vi "post_processing.vi"(4 "wl end":dbl, 6 "wl start":dbl, 7 "Phase warning":dbl, 8 "Wavelengths":dbl[](array[numeric]), 9 "Phase in (r=wl, c=v)":dbl[][](array[numeric]), 10 "Zeroes (idx)":cluster{"Splice indices":i32[]}[](array[cluster]), 11 "Extrapolate":bool) -> (0 "Phase out (r=wl, c=v)":dbl[][](array[numeric]), 3 "Errors":T1)   [LabVIEW 2019]
uses:
  <vilib>/gmath/NI_Gmath.lvlib
panel:
  out "max 2nd deriv":dbl
  out "d2/dV2 Phase":dbl[](array[numeric])
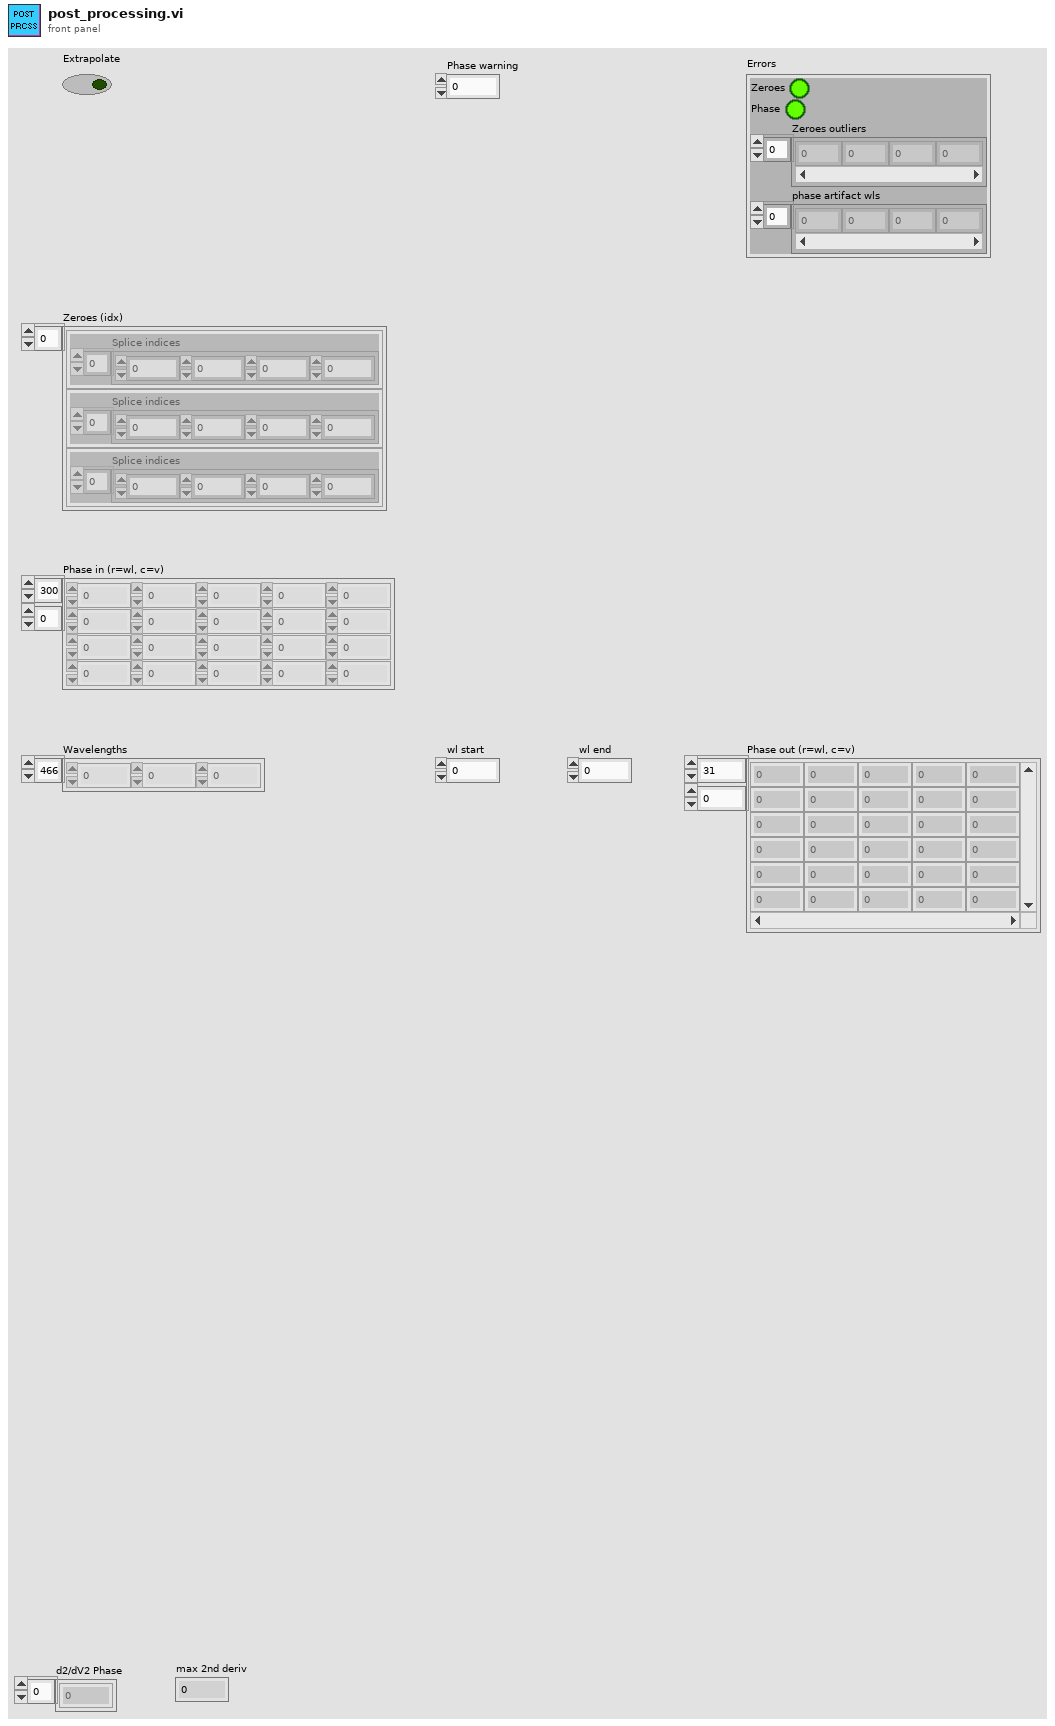
[diagram p1: front panel]
types:
  T1 = cluster{"Zeroes":bool, "Phase":bool, "Zeroes outliers":dbl[], "phase artifact wls":dbl[]}
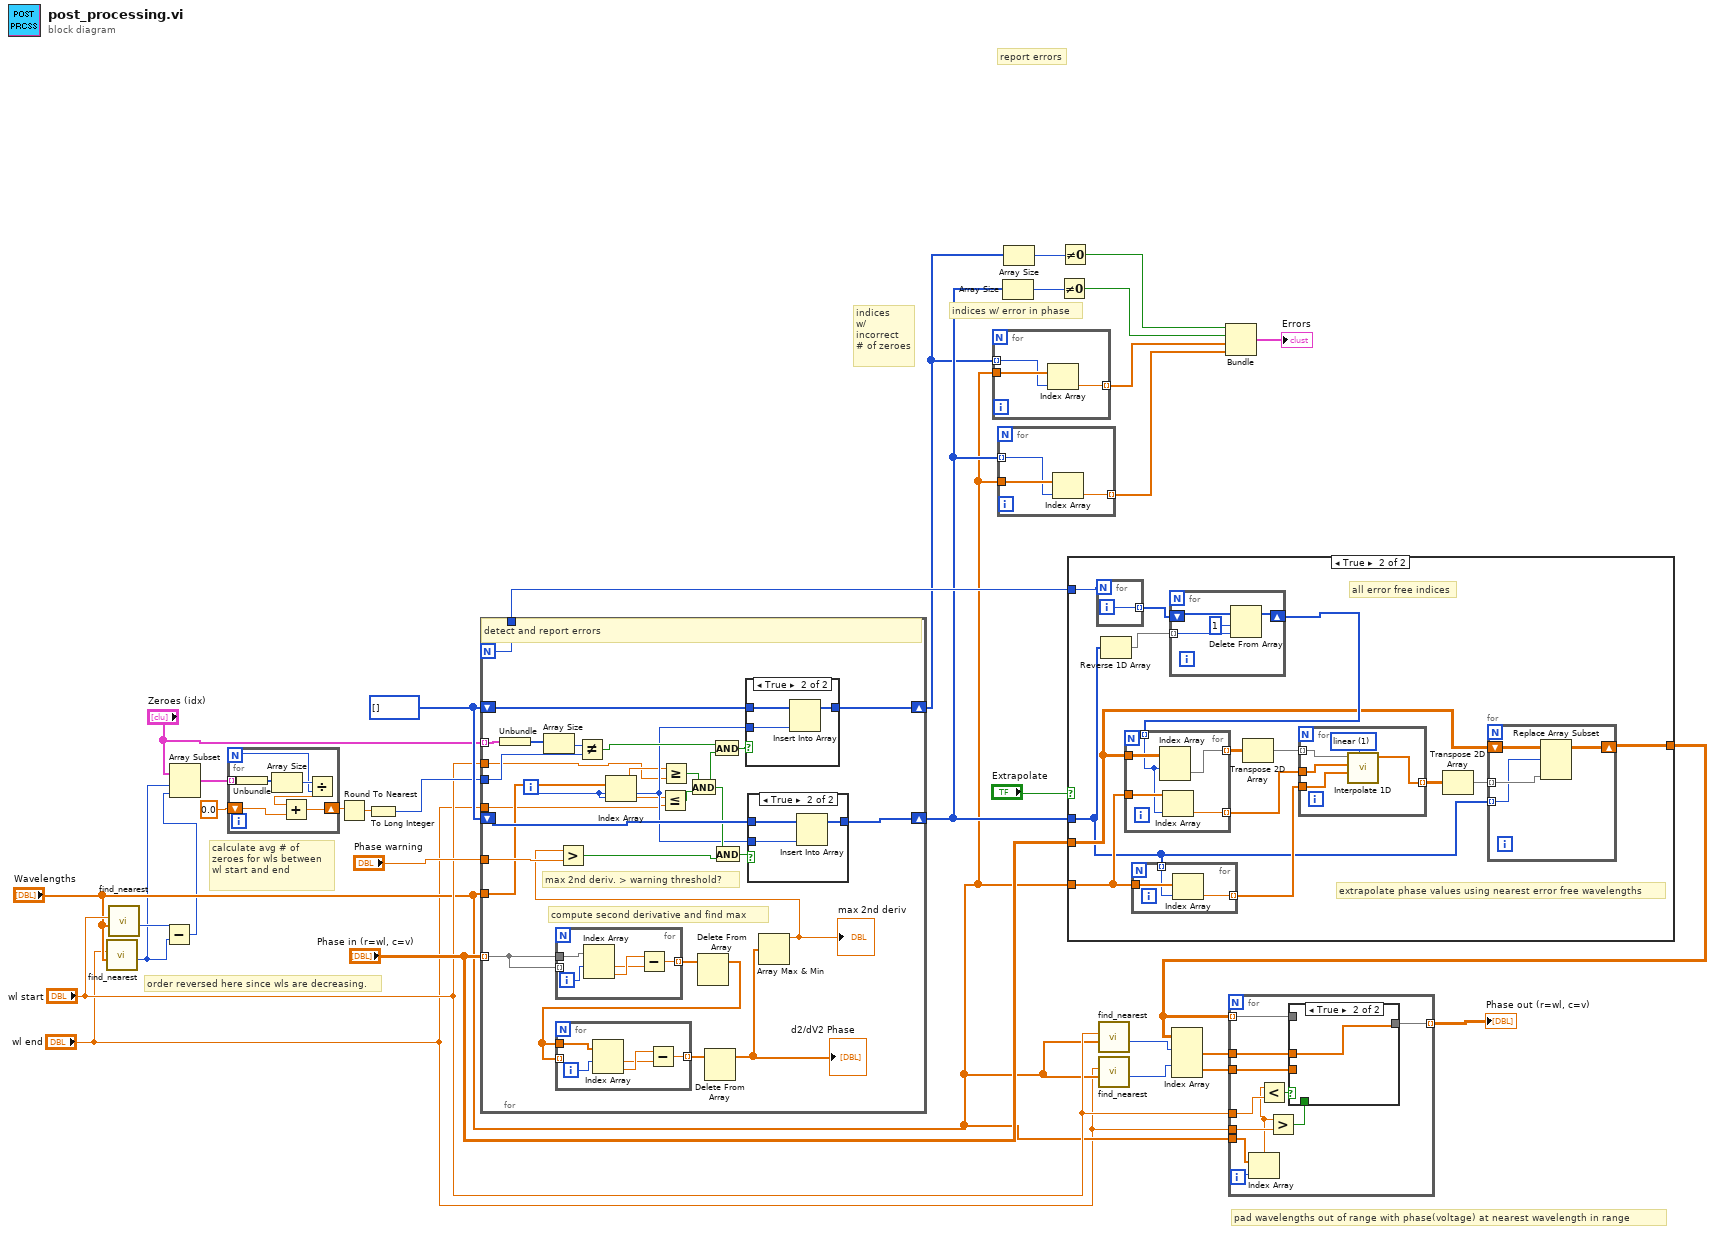
[diagram p0: block diagram]
diagram:
  w32 = i32[] []
  # "calculate avg # of zeroes for wls between wl start and end"
  # "order reversed here since wls are decreasing."
  # "indices w/ error in phase"
  # "indices\nw/\nincorrect\n# of zeroes"
  # "report errors"
  # "pad wavelengths out of range with phase(voltage) at nearest wavelength in range"
  n1 = call "find_nearest.vi"("Sorted Array (<)"="Wavelengths", "Key"="wl end") -> ("Nearest index"=w2:i32)  [unwired: 6 in, 3 out]
  n2 = call "find_nearest.vi"("Sorted Array (<)"="Wavelengths", "Key"="wl start") -> ("Nearest index"=w3:i32)  [unwired: 6 in, 3 out]
  n3 = Subtract(x=w3, y=w2) -> (x-y=w1:i32)
  n4 = Array Subset(array="Zeroes (idx)", index=w2, length=w1) -> (w5:cluster{"Splice indices":i32[]}[])
  n5 = for {
    N -> [w36]
    tunnel: w5 -> [w38] mode=indexing
    shift-right: [w33] -> w11
    shift-left: 0.0 -> [w35]
    n6 = Unbundle(w38) -> ("Splice indices"=w39:i32[])
    n7 = Array Size(array=w39) -> (size(s)=w37:i32)
    n8 = Divide(x=w37, y=w36) -> (x/y=w34:dbl)
    n9 = Add(x=w34, y=w35) -> (x+y=w33:dbl)
  }
  n10 = Round To Nearest(number=w11) -> (nearest integer value=w10:dbl)
  n11 = To Long Integer(number=w10) -> (32bit integer=w9:i32)
  n12 = for {
    N -> [w54]
    shift-right: [w66] -> w22
    shift-left: w32 -> [w67]
    shift-right: [w63] -> w21
    shift-left: w32 -> [w64]
    tunnel: w9 -> [w62]
    tunnel: "Phase warning" -> [w61]
    tunnel: "Zeroes (idx)" -> [w43] mode=indexing
    tunnel: "Phase in (r=wl, c=v)" -> [w57] mode=indexing
    tunnel: [w54] -> w29
    tunnel: "Wavelengths" -> [w45]
    tunnel: "wl start" -> [w41]
    tunnel: "wl end" -> [w40]
    i -> [w46]
    # "max 2nd deriv. > warning threshold?"
    # "compute second derivative and find max"
    # "detect and report errors"
    n13 = Unbundle(w43) -> ("Splice indices"=w42:i32[])
    n14 = Array Size(array=w42) -> (size(s)=w65:i32)
    n15 = for {
      tunnel: w57 -> [w75]
      tunnel: [w73] -> w58 mode=indexing
      tunnel: w57 -> [_] mode=indexing
      i -> [w77]
      n16 = Index Array(array=w75, index #1=w77) -> (element #1=w74:dbl, element #2=w76:dbl)  [unwired: 1 in]
      n17 = Subtract(x=w76, y=w74) -> (x-y=w73:dbl)
    }
    n18 = Not Equal?(x=w65, y=w62) -> (x != y?=w51:bool)
    n19 = Index Array(array=w45, index=w46) -> (element=w44:dbl)
    n20 = Less Or Equal?(x=w44, y=w40) -> (x <= y?=w53:bool)
    n21 = Greater Or Equal?(x=w44, y=w41) -> (x >= y?=w52:bool)
    n22 = And(x=w52, y=w53) -> (x .and. y?=w47:bool)
    n23 = Delete From Array(array=w58) -> (array with subset deleted=w56:dbl[])  [unwired: 2 in, 1 out]
    n24 = for {
      tunnel: w56 -> [w70]
      tunnel: [w68] -> w59 mode=indexing
      tunnel: w56 -> [_] mode=indexing
      i -> [w72]
      n25 = Index Array(array=w70, index #1=w72) -> (element #1=w69:dbl, element #2=w71:dbl)  [unwired: 1 in]
      n26 = Subtract(x=w71, y=w69) -> (x-y=w68:dbl)
    }
    n27 = Delete From Array(array=w59) -> (array with subset deleted=w60:dbl[])  [unwired: 2 in, 1 out]
    "d2/dV2 Phase" <- w60
    n28 = And(x=w51, y=w47) -> (x .and. y?=w50:bool)
    n29 = case shown="True" w50 {
      tunnel: w46 -> [_ w80]
      tunnel: w64 -> [w78 w81]
      tunnel: [w78 w79] -> w63
      frame False {
      }
      frame True {
        n30 = Insert Into Array(array=w81, new element=w80) -> (w79:i32[])  [unwired: 1 in]
      }
    }
    n31 = Array Max & Min(array=w60) -> (max value=w55:dbl)  [unwired: 3 out]
    "max 2nd deriv" <- w55
    n32 = Greater?(x=w55, y=w61) -> (0:w49:bool)
    n33 = And(x=w47, y=w49) -> (x .and. y?=w48:bool)
    n34 = case shown="True" w48 {
      tunnel: w46 -> [_ w84]
      tunnel: w67 -> [w82 w85]
      tunnel: [w82 w83] -> w66
      frame False {
      }
      frame True {
        n35 = Insert Into Array(array=w85, new element=w84) -> (w83:i32[])  [unwired: 1 in]
      }
    }
  }
  n36 = for {
    tunnel: w21 -> [w87] mode=indexing
    tunnel: "Wavelengths" -> [w88]
    tunnel: [w86] -> w18 mode=indexing
    n37 = Index Array(array=w88, index=w87) -> (element=w86:dbl)
  }
  n38 = for {
    tunnel: w22 -> [w90] mode=indexing
    tunnel: "Wavelengths" -> [w91]
    tunnel: [w89] -> w17 mode=indexing
    n39 = Index Array(array=w91, index=w90) -> (element=w89:dbl)
  }
  n40 = Array Size(array=w22) -> (size(s)=w24:i32)
  n41 = Array Size(array=w21) -> (size(s)=w23:i32)
  n42 = Not Equal To 0?(x=w24) -> (x != 0?=w19:bool)
  n43 = Not Equal To 0?(x=w23) -> (x != 0?=w20:bool)
  n44 = case shown="True" "Extrapolate" {
    tunnel: "Phase in (r=wl, c=v)" -> [w92 w98]
    tunnel: [w92 w95] -> w15
    tunnel: w29 -> [_ w106]
    tunnel: w22 -> [_ w96]
    tunnel: "Wavelengths" -> [_ w103]
    frame False {
    }
    frame True {
      # "extrapolate phase values using nearest error free wavelengths"
      # "all error free indices"
      n45 = for {
        N: w106 -> [_]
        tunnel: [w111] -> w94 mode=indexing
        i -> [w111]
      }
      n46 = Reverse 1D Array(array=w96) -> (reversed array=w93:i32[])
      n47 = for {
        tunnel: w103 -> [w123]
        tunnel: [w122] -> w100 mode=indexing
        tunnel: w96 -> [w121] mode=indexing
        n48 = Index Array(array=w123, index=w121) -> (element=w122:dbl)
      }
      n49 = for {
        shift-right: [w109] -> w105
        shift-left: w94 -> [w110]
        tunnel: w93 -> [w108] mode=indexing
        n50 = Delete From Array(array=w110, length=1, index=w108) -> (array with subset deleted=w109:i32[])  [unwired: 1 out]
      }
      n51 = for {
        tunnel: w98 -> [w128]
        tunnel: w105 -> [w125] mode=indexing
        tunnel: [w127] -> w104 mode=indexing
        tunnel: w103 -> [w126]
        tunnel: [w124] -> w101 mode=indexing
        n52 = Index Array(array=w128, index (row)=w125) -> (element=w127:dbl[])  [unwired: 1 in]
        n53 = Index Array(array=w126, index=w125) -> (element=w124:dbl)
      }
      n54 = Transpose 2D Array(2D array=w104) -> (transposed array=w102:dbl[][])
      n55 = for {
        tunnel: w102 -> [w120] mode=indexing
        tunnel: w101 -> [w119]
        tunnel: w100 -> [w118]
        tunnel: [w116] -> w99 mode=indexing
        w117 = 1 items=["nearest", "linear", "spline", "cubic Hermite", "Lagrange"] ("method")
        n56 = call <vilib>:"Interpolate 1D.vi"("method"=w117, "xi"=w118, "X"=w119, "Y"=w120) -> ("yi"=w116:dbl[])  [unwired: 5 in, 2 out]
      }
      n57 = Transpose 2D Array(2D array=w99) -> (transposed array=w97:dbl[][])
      n58 = for {
        tunnel: w97 -> [w114] mode=indexing
        tunnel: w96 -> [w113] mode=indexing
        shift-right: [w112] -> w95
        shift-left: w98 -> [w115]
        n59 = Replace Array Subset(array=w115, new element=w114, index (row)=w113) -> (w112:dbl[][])  [unwired: 1 in]
      }
    }
  }
  n60 = call "find_nearest.vi"("Sorted Array (<)"="Wavelengths", "Key"="wl start") -> ("Nearest index"=w13:i32)  [unwired: 6 in, 3 out]
  n61 = call "find_nearest.vi"("Sorted Array (<)"="Wavelengths", "Key"="wl end") -> ("Nearest index"=w14:i32)  [unwired: 6 in, 3 out]
  n62 = Index Array(array=w15, index (row) #1=w13, index (row) #2=w14) -> (element #1=w27:dbl[], element #2=w26:dbl[])  [unwired: 2 in]
  n63 = Bundle(w20, w19, w18, w17) -> (→"Errors":cluster{bool, bool, dbl[], dbl[]})  [unwired: 1 in]
  n64 = for {
    tunnel: w15 -> [w133] mode=indexing
    tunnel: "wl start" -> [w139]
    tunnel: "wl end" -> [w137]
    tunnel: w27 -> [w135]
    tunnel: w26 -> [w134]
    tunnel: [w132] -> w25 mode=indexing
    tunnel: "Wavelengths" -> [w131]
    i -> [w130]
    n65 = Index Array(array=w131, index=w130) -> (element=w129:dbl)
    n66 = Less?(x=w129, y=w139) -> (x < y?=w138:bool)
    n67 = Greater?(x=w129, y=w137) -> (0:w136:bool)
    n68 = case shown="True" w138 {
      tunnel: w136 -> [w143 _]
      tunnel: w135 -> [_ w146]
      tunnel: w134 -> [w142 _]
      tunnel: w133 -> [w141 _]
      tunnel: [w140 w146] -> w132
      frame False {
        n69 = case shown="False" w143 {
          tunnel: [w144 w145] -> w140
          tunnel: w142 -> [_ w145]
          tunnel: w141 -> [w144 _]
          frame False {
          }
          frame True {
          }
        }
      }
      frame True {
      }
    }
  }
  "Phase out (r=wl, c=v)" <- w25
